vi "macro_AngleStats_AngleAdd_CallbackHelp.vi"   [LabVIEW 2019, in "Trajectory_Library.lvlib"]
uses:
  Trajectory_Library.lvlib
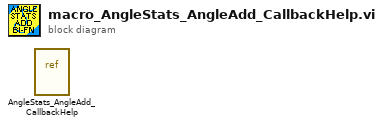
[diagram p0: block diagram]
diagram:
  n1 = vi-ref "AngleStats_AngleAdd_CallbackHelp.vi"() -> ()  [unwired: 1 out]
